vi "ActTurn.vi"(9 "FirstTime":bool, 10 "MaxSpeed (ft/s)":dbl, 11 "Degrees":dbl) -> (0 "RotationSpeedDemand Deg/Sec":dbl, 3 "Done":bool)   [LabVIEW 2023]
doc: "Robot will turn a set number of degrees utilizing position control \n\nInputs:\n-- MaxSpeed -- Double -- In ft/s, the MaxSpeed the robot can go -- \n-- Degrees -- Double -- Rotation in degrees you want the robot to go -- \n-- FirstTime -- Boolean -- Input true the first time this function is called, sets the target position -- \n\nOutputs:\n-- Done -- Bool -- has the robot reached its target distance -- \n-- LeftSpeedDemand -- Double -- Speed Demand for left drive train inorder to reach target -- \n-- RightSpeedDemand -- Double -- Speed Demand for left drive train inorder to reach target --"
uses:
  <vilib>/Rock Robotics/WPI/ThirdParty/JAS_Junk/TrajLib/Trajectory_Library.lvlib
  <vilib>/Rock Robotics/Network Tables/NT Write Number.vi
  <vilib>/Rock Robotics/Network Tables/NT Write Boolean.vi
panel:
  out "Unfiltetred Done":bool
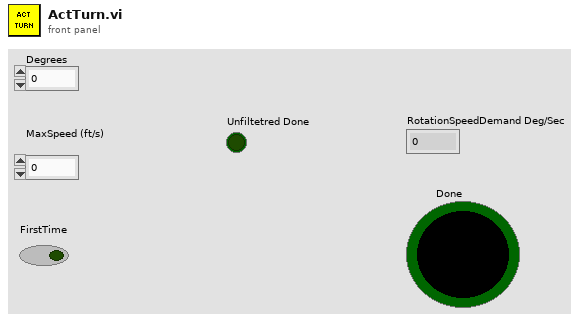
[diagram p1: front panel]
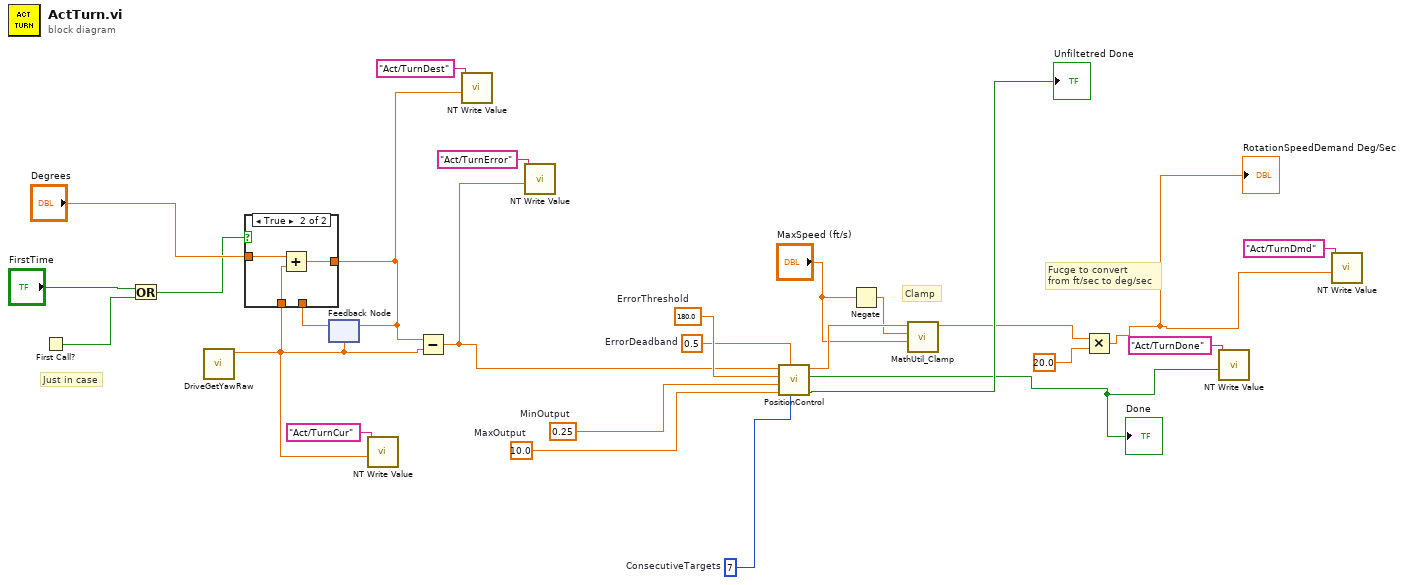
[diagram p0: block diagram]
diagram:
  w17 = 10.0  # MaxOutput
  w18 = 0.25  # MinOutput
  w22 = 7  # ConsecutiveTargets
  w23 = 0.5  # ErrorDeadband
  w24 = 180.0  # ErrorThreshold
  # "Just in case"
  # "Fucge to convert\nfrom ft/sec to deg/sec"
  # "Clamp"
  n1 = First Call?() -> (First Call?: T/F=w2:bool)
  n2 = Or(x="FirstTime", y=w2) -> (x .or. y?=w1:bool)
  n3 = call "DriveGetYawRaw.vi"() -> ("YawRaw"=w4:dbl)  [unwired: 11 in]
  n4 = feedback #1(w4) -> (w25:dbl)
  n5 = case shown="True" w1 {
    tunnel: "Degrees" -> [_ w30]
    tunnel: [w27 w29] -> w6
    tunnel: w25 -> [w27 _]
    tunnel: w4 -> [_ w28]
    frame False {
    }
    frame True {
      n6 = Add(x=w30, y=w28) -> (x+y=w29:dbl)
    }
  }
  n7 = feedback-in #1(w6) -> ()
  n8 = call-poly <vilib>:"NT Write Value.vi"("value"=w4, "name"="Act/TurnCur") -> ()  [unwired: 9 in, 1 out]
  n9 = Subtract(x=w6, y=w4) -> (x-y=w14:dbl)
  n10 = call-poly <vilib>:"NT Write Value.vi"("value"=w6, "name"="Act/TurnDest") -> ()  [unwired: 9 in, 1 out]
  n11 = call-poly <vilib>:"NT Write Value.vi"("value"=w14, "name"="Act/TurnError") -> ()  [unwired: 9 in, 1 out]
  n12 = call "PositionControl.vi"("ConsecutiveTargets"=w22, "ErrorDeadband"=w23, "MaxOutput"=w17, "MinOutput"=w18, "ErrorThreshold"=w24, "Error"=w14) -> ("UnfilteredOnTarget"=→"Unfiltetred Done":bool, "OnTarget"=w12:bool, "OutputValue"=w21:dbl)  [unwired: 3 in]
  "Done" <- w12
  n13 = Negate(x="MaxSpeed (ft/s)") -> (-x=w20:dbl)
  n14 = call <vilib>:"MathUtil_Clamp.vi"("High Limit"="MaxSpeed (ft/s)", "Low Limit"=w20, "Value"=w21) -> ("Result"=w10:dbl)  [unwired: 8 in]
  n15 = Multiply(x=w10, y=20.0) -> (x*y=w8:dbl)
  "RotationSpeedDemand Deg/Sec" <- w8
  n16 = call-poly <vilib>:"NT Write Value.vi"("value"=w12, "name"="Act/TurnDone") -> ()  [unwired: 9 in, 1 out]
  n17 = call-poly <vilib>:"NT Write Value.vi"("value"=w8, "name"="Act/TurnDmd") -> ()  [unwired: 9 in, 1 out]
